vi "Add uSs from Run Config.vi"(8 "error in (no error)":errorcluster, 10 "uS List":string[](array[string]), 11 "Guardian in":refnum<class "Guardian.lvclass">) -> (0 "error out":errorcluster, 3 "Guardian out":refnum<class "Guardian.lvclass">)   [LabVIEW 2026, in "TALOS.lvlib" / "Guardian.lvlib" / "Guardian.lvclass"]
uses:
  Guardian.lvclass
  C:/LabVIEW Code/TALOS/builds/Actor Framework PPL/Actor Framework.lvlibp/1abvi3w/vi.lib/ActorFramework/Actor/Actor.lvclass
  Classes/uService List/uService List.lvclass/uService List.ctl
  Guardian Messages/Launch uService Msg/Launch uService Msg.lvclass/Launch uService Msg.ctl
  Ancestor/Ancestor/Ancestor.lvclass/Ancestor.ctl
  Classes/uService List/Get all IDs.vi
  fcb3572a-2cec-4fc7-ae89-858ca11508d7.vi
  Support VIs/Generate Error.vi
  FGV/Error Memory/Get Error Description.vi
  Support VIs/Get PC name.vi
  Ancestor/Ancestor/Read ID.vi
  Support VIs/Get Class Name.vi
  <vilib>/Utility/error.llb/Clear Errors.vi
  FGV/Error Memory/Error Memory Core.vi
  <vilib>/AdvancedString/Delimited String to 1D String Array.vi
  <vilib>/AdvancedString/Delimited String to 1D String Array (string).vi
  Support VIs/Circus Root Path.vi
  FGV/Error Memory/Error Crt Lvl checker.vi
  FGV/Error Memory/Error Memory Core.vi/40c8088d-b597-4017-91af-faa98e00292e.vi
  FGV/Error Memory/Error Memory Core.vi/d4a3ab98-063c-4e44-b43d-fbdcfe6c2be2.vi
  builds/Actor Framework PPL/Actor Framework.lvlibp/1abvi3w/vi.lib/ActorFramework/Message Enqueuer/Enqueue.vi
  Support VIs/Global Memory.vi
  <vilib>/Utility/LVClass/Get LV Class Name.vi
  Support VIs/Is in Packed Library.vi
  Support VIs/TALOS Root path.vi
  Support VIs/Read CSV worksheet.vi
  Support VIs/Global Constants.vi
  <vilib>/Utility/error.llb/General Error Handler.vi
  Support VIs/Error Log.vi
  Guardian Messages/Launch uService Msg/Launch uService Msg.lvclass
  Guardian Messages/I am alive Msg/I am alive Msg.lvclass
  Ancestor/Ancestor/Ancestor.lvclass
  <vilib>/Comparison/Equal/Equal Functor/Equal Functor.lvclass
  Classes/uService List/uService List.lvclass
  builds/Actor Framework PPL/Actor Framework.lvlibp/1abvi3w/vi.lib/ActorFramework/Actor/Actor.lvclass
  TALOS.lvlib
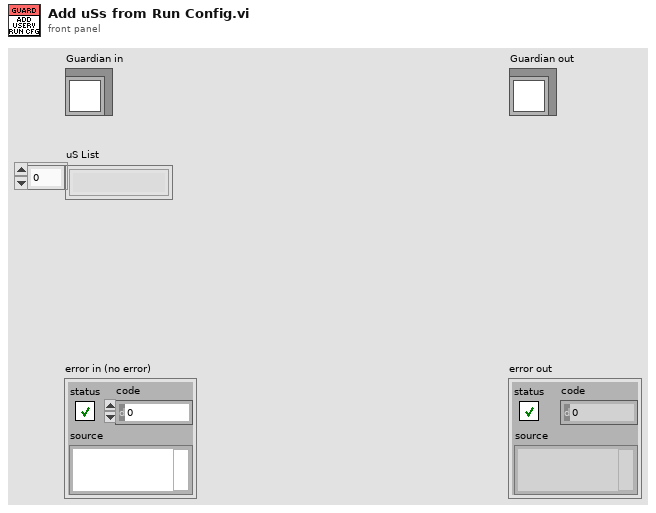
[diagram p1: front panel]
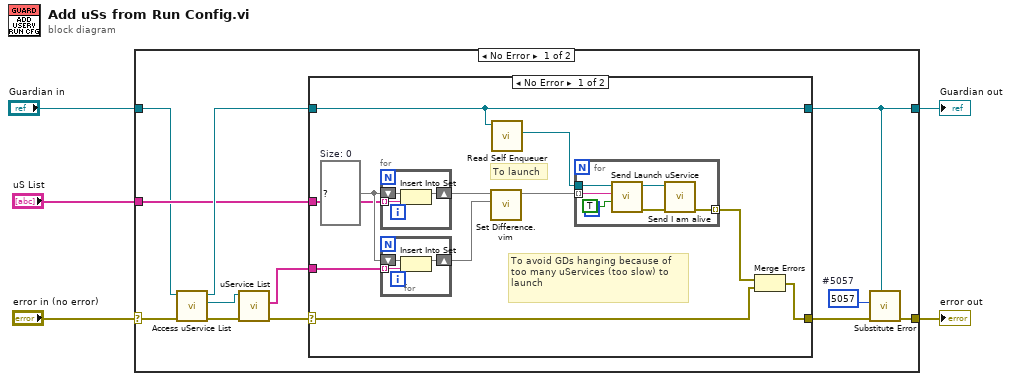
[diagram p0: block diagram]
diagram:
  n1 = case shown="No Error" "error in (no error)" {
    selector: "error in (no error)" -> [w8 w44]
    tunnel: [w11 w44] -> w4
    tunnel: [w10 w43] -> w2
    tunnel: "Guardian in" -> [w6 w43]
    tunnel: "uS List" -> [w7 _]
    frame No Error {
      w9 = 5057  # #5057
      n2 = call-dynamic "Access uService List.vi"("error in (no error)"=w8, "Ancestor in"=w6) -> ("error out"=w16:errorcluster, "uService List out"=w17:refnum<class "uService List.lvclass">, "Ancestor out"=w14:refnum<class "Guardian.lvclass">)  [unwired: 7 in]
      n3 = call-poly "uService List.vi"("error in (no error)"=w16, "uService List"=w17) -> ("error out"=w13:errorcluster, "All IDs"=w15:string[])  [unwired: 7 in, 1 out]
      n4 = case shown="No Error" w13 {
        selector: w13 -> [w19 w42]
        tunnel: w7 -> [w26 _]
        tunnel: w15 -> [w24 _]
        tunnel: w14 -> [w22 w41]
        tunnel: [w18 w42] -> w12
        tunnel: [w22 w41] -> w10
        frame No Error {
          w27 = set{string} {}  # Size: 0
          # "To avoid GDs hanging because of too many uServices (too slow) to launch"
          # "To launch"
          n5 = for {
            shift-right: [w34] -> w25
            shift-left: w27 -> [w33]
            tunnel: w26 -> [w32] mode=indexing
            n6 = Insert Into Set(10:w32, 11:w33) -> (3:w34:set{string})  [unwired: 1 out]
          }
          n7 = for {
            shift-right: [w31] -> w23
            shift-left: w27 -> [w30]
            tunnel: w24 -> [w29] mode=indexing
            n8 = Insert Into Set(10:w29, 11:w30) -> (3:w31:set{string})  [unwired: 1 out]
          }
          n9 = call "Set Difference.vim"("set 2"=w23, "set 1"=w25) -> ("difference"=w28:set{string})  [unwired: 9 in]
          n10 = call "Read Self Enqueuer.vi"("Actor"=w22) -> ("Self Enqueuer"=w21:refnum<class "Message Enqueuer.lvclass">)  [unwired: 10 in]
          n11 = for {
            tunnel: w28 -> [w39] mode=indexing
            tunnel: w21 -> [w40]
            tunnel: [w36] -> w20 mode=indexing
            n12 = call "Send Launch uService.vi"("GUI?"=TRUE, "uService Class Name"=w39, "Message Enqueuer"=w40) -> ("error out"=w37:errorcluster, "Message Enqueuer out"=w35:refnum<class "Message Enqueuer.lvclass">)  [unwired: 7 in]
            n13 = call "Send I am alive.vi"("error in (no error)"=w37, "Message Enqueuer"=w35) -> ("error out"=w36:errorcluster)  [unwired: 8 in, 1 out]
          }
          n14 = Merge Errors(w20, w19) -> (w18:errorcluster)
        }
        frame Error {
        }
      }
      n15 = call "Substitute Error.vi"("LabVIEW Object"=w10, "error in (no error)"=w12, "Error Code"=w9) -> ("error out"=w11:errorcluster)  [unwired: 8 in]
    }
    frame Error {
    }
  }
  "error out" <- w4
  "Guardian out" <- w2
